vi "Check_Trigger_and_run.vi"(7 "DAQ_VI":refnum<vi>, 8 "error in (no error)":errorcluster, 10 "Command_Message_in":T1, 11 "Command_queue_in":T2) -> (0 "error out":errorcluster, 2 "Command_Message_out":T1)   [LabVIEW 2019]
uses:
  Command_Message.ctl
  Command_Queue.ctl
panel:
  out "everyting okay?":bool
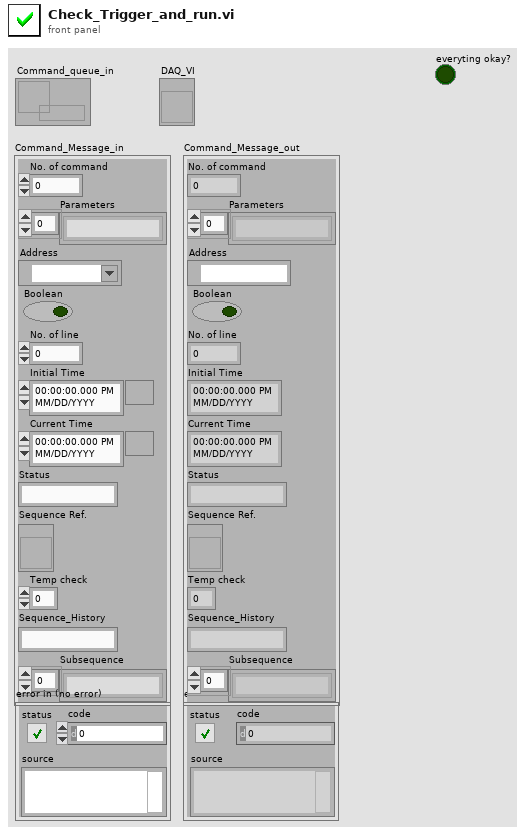
[diagram p1: front panel]
types:
  T1 = typedef "Command_Message.ctl" = cluster{"No. of command":i32, "Parameters":string[], "Address":refnum<visa-resource-name>, "Boolean":bool, "No. of line":i32, "Initial Time":timestamp, "Current Time":timestamp, "Status":string, "Sequence Ref.":refnum<vi>, "Temp check":i32, "Sequence_History":string, "Subsequence":string[]}
  T2 = typedef "Command_Queue.ctl" = refnum<queue>
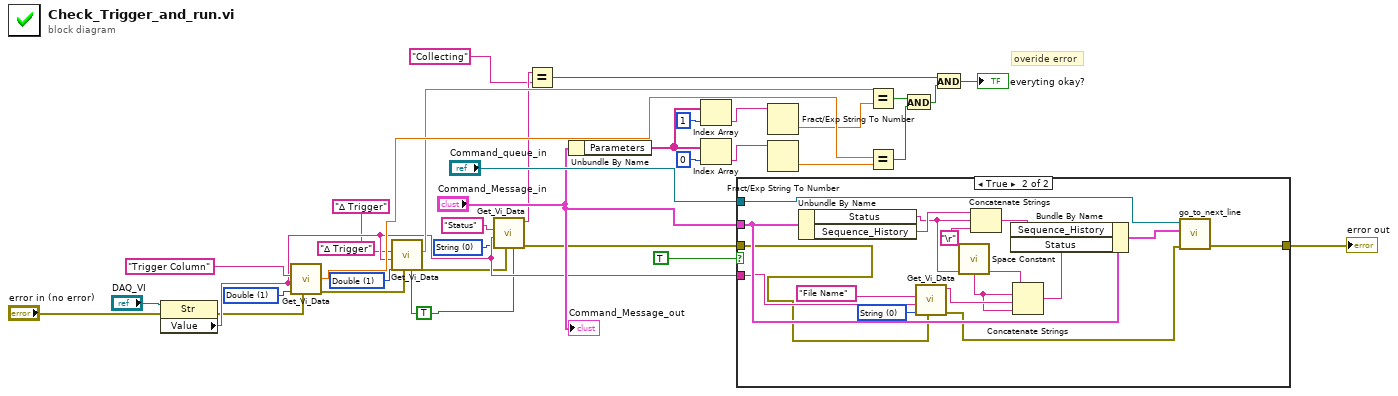
[diagram p0: block diagram]
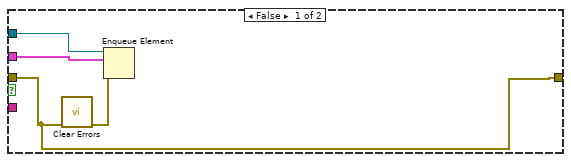
[diagram p2: hidden frame]
diagram:
  w2 = TRUE ("bypass")
  w12 = u16 0 items=["String", "Double", "Boolean", "Variant"] ("Data Type")
  w32 = u16 1 items=["String", "Double", "Boolean", "Variant"] ("Data Type")
  (unwired) "∆ Trigger"
  w34 = u16 1 items=["String", "Double", "Boolean", "Variant"] ("Data Type")
  # "overide error"
  n1 = property on="Property Node" class="Str"(reference="DAQ_VI", error in="error in (no error)") -> (error out=w6:errorcluster, "Value"=w15:string)  [unwired: 1 out]
  n2 = call "Get_Vi_Data.vi"("error in (no error) 2"=w6, "Data Type"=w34, "VI name"=w15, "Control Name"="Trigger Column") -> ("error out"=w16:errorcluster, "Data (Double)"=w28:dbl)  [unwired: 3 in, 3 out]
  n3 = call "Get_Vi_Data.vi"("bypass"=w2, "error in (no error) 2"=w16, "Data Type"=w32, "VI name"=w15, "Control Name"="∆ Trigger") -> ("error out"=w13:errorcluster, "Data (Double)"=w25:dbl)  [unwired: 2 in, 3 out]
  n4 = call "Get_Vi_Data.vi"("bypass"=w2, "error in (no error) 2"=w13, "Data Type"=w12, "VI name"=w15, "Control Name"="Status") -> ("error out"=w3:errorcluster, "Data (String)"=w11:string)  [unwired: 2 in, 3 out]
  n5 = Equal?(x=w11, y="Collecting" ("Data (String)")) -> (x = y?=w9:bool)
  n6 = Unbundle By Name("Command_Message_in") -> ("Parameters"=w18:string[])
  n7 = Index Array(array=w18, index=1) -> (element=w29:string)
  n8 = Index Array(array=w18, index=0) -> (element=w27:string)
  n9 = case shown="True" TRUE {
    tunnel: "Command_queue_in" -> [w38 w49]
    tunnel: "Command_Message_in" -> [w37 w54]
    tunnel: w3 -> [w35 w40]
    tunnel: [w35 w53] -> w20
    tunnel: w15 -> [_ w48]
    frame False {
      n10 = call <vilib>:"Clear Errors.vi"("error in (no error)"=w35) -> ("error out"=w36:errorcluster)  [unwired: 5 in, 1 out]
      n11 = Enqueue Element(queue=w38, element=w37, error in (no error)=w36) -> ()  [unwired: 1 in, 3 out]
    }
    frame True {
      w46 = u16 0 items=["String", "Double", "Boolean", "Variant"] ("Data Type")
      n12 = Unbundle By Name(w54) -> ("Status"=w44:string, "Sequence_History"=w50:string)
      n13 = call "Get_Vi_Data.vi"("error in (no error) 2"=w40, "Data Type"=w46, "VI name"=w48, "Control Name"="File Name") -> ("error out"=w39:errorcluster, "Data (String)"=w43:string)  [unwired: 3 in, 3 out]
      n14 = call <vilib>:"Space Constant.vi"() -> ("String"=w42:string)
      n15 = Concatenate Strings(w50, w44, "\r") -> (w51:string)
      n16 = Concatenate Strings(w44, w42, w43, w42) -> (w41:string)
      n17 = Bundle By Name(cluster=w54, "Sequence_History"=w51, "Status"=w41) -> (w52:T1)
      n18 = call "go_to_next_line.vi"("error in (no error)"=w39, "Message_command in"=w52, "Command Queue in"=w49) -> ("error out"=w53:errorcluster)  [unwired: 7 in, 1 out]
    }
  }
  "error out" <- w20
  n19 = Fract/Exp String To Number(string=w29) -> (number=w24:dbl)  [unwired: 3 in, 1 out]
  n20 = Fract/Exp String To Number(string=w27) -> (number=w26:dbl)  [unwired: 3 in, 1 out]
  n21 = Equal?(x=w25, y=w24) -> (x = y?=w23:bool)
  n22 = Equal?(x=w28, y=w26) -> (x = y?=w22:bool)
  n23 = And(x=w23, y=w22) -> (x .and. y?=w8:bool)
  n24 = And(x=w9, y=w8) -> (x .and. y?=→"everyting okay?":bool)
  "Command_Message_out" <- "Command_Message_in"
